vi "practice05_sync_raw.vi"() -> ()   [LabVIEW 2025]
uses:
  <vilib>/Instr/_visa.llb/VISA Configure Serial Port (Instr).vi
  <vilib>/express/express arith-compare/Formula/XNode/ExpressFormulaBlockNode.xnode
panel:
  in  "Pin Analogico":string(combo)="0"
  out "Voltaje 2":dbl
  out "Voltaje":dbl(graph)
  in  "stop":bool
  in  "Muestreo":u32
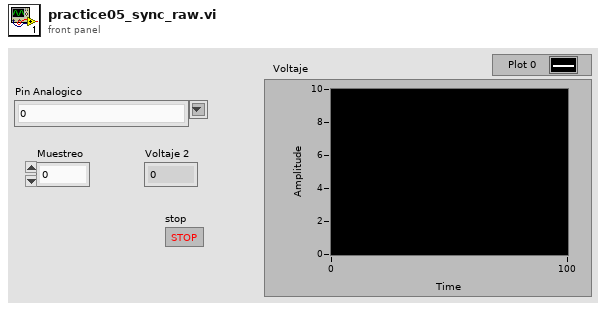
[diagram p1: front panel]
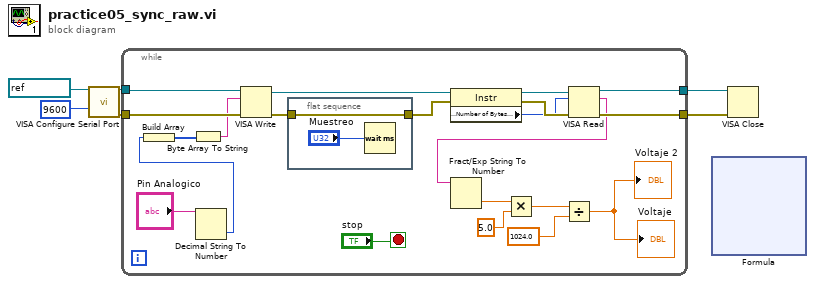
[diagram p0: block diagram]
diagram:
  n1 = call-poly "VISA Configure Serial Port"("VISA resource name"=refnum<visa-resource-name> "COM3", "parity (0:none)"=9600) -> ("VISA resource name out"=w4:refnum<visa-resource-name>, "error out"=w3:errorcluster)  [unwired: 12 in]
  n2 = while {
    tunnel: w4 -> [w22]
    tunnel: w3 -> [w21]
    tunnel: [w26] -> w2
    tunnel: [w23] -> w1
    stop <- "stop" stop-if-true
    n3 = Decimal String To Number(string="Pin Analogico") -> (number=w8:i32)  [unwired: 2 in, 1 out]
    n4 = Build Array(w8) -> (w7:i32[])
    n5 = Byte Array To String(unsigned byte array=w7) -> (string=w10:string)
    n6 = VISA Write(VISA resource name=w22, write buffer=w10, error in (no error)=w21) -> (VISA resource name out=w20:refnum<visa-resource-name>, error out=w19:errorcluster)  [unwired: 1 out]
    n7 = flat-sequence {
      tunnel: w19 -> [w28]
      tunnel: [w28] -> w18
      frame #0 {
        n8 = Wait (ms)(milliseconds to wait="Muestreo") -> ()  [unwired: 1 out]
      }
    }
    n9 = property class="Instr"(reference=w20, error in=w18) -> (reference out=w25:refnum<visa-resource-name>, error out=w24:errorcluster, "Serial Settings:Number of Bytes at Serial Port"=w17:u32)
    n10 = VISA Read(VISA resource name=w25, byte count=w17, error in (no error)=w24) -> (VISA resource name out=w26:refnum<visa-resource-name>, read buffer=w16:string, error out=w23:errorcluster)  [unwired: 1 out]
    n11 = Fract/Exp String To Number(string=w16) -> (number=w15:dbl)  [unwired: 3 in, 1 out]
    n12 = Multiply(x=w15, y=5.0) -> (x*y=w13:dbl)
    n13 = Divide(x=w13, y=1024.0) -> (x/y=→"Voltaje" →"Voltaje 2":dbl)
  }
  n14 = xnode "Formula"() -> ()  [unwired: 2 in, 2 out]
  n15 = VISA Close(VISA resource name=w2, error in (no error)=w1) -> ()  [unwired: 1 out]
